vi "RS 485 IO.vi"(6 "Port":T1, 10 "Input in":T2={"Data"=[0, 0, 0, 0, 0, 0, 0, 0, 0, 0, 0, 0, 0, 0, 0, 0, 0, 0, 0, 0], "NumBytes"=0, "RS485_Cmd"=enum."Read", "Timeout (ms)"=0}) -> (3 "Input out":T3)   [LabVIEW 2015]
uses:
  RS485 In.ctl
  Serial Data In.ctl
  Port.ctl
  <vilib>/rvi/Emulation/niFpgaGetClockAttributes.vi
  <vilib>/rvi/Emulation/niFpgaSctlEmulationGetInTimedLoop.vi
  <vilib>/rvi/Emulation/niFpgaEmulationReportErrorSimple.vi
  <vilib>/rvi/eio/common/nirviEmuTemplateMethod_errors.vi
  <vilib>/rvi/Emulation/niFpgaCriticalErrorInLSC.vi
  <vilib>/eio/EIOMethodNode/EIOMethodNode.xnode
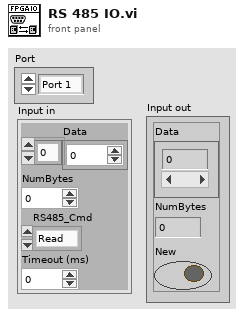
[diagram p1: front panel]
types:
  T1 = typedef "Port.ctl" = enum8{"Port 1", "Port 2", "Port 3", "Port 4", "None"}
  T2 = typedef "Serial Data In.ctl" = cluster{"Data":u8[], "NumBytes":i32, "RS485_Cmd":enum8{"Read", "Write", "Idle"}, "Timeout (ms)":i32}
  T3 = typedef "RS485 In.ctl" = cluster{"Data":u8[], "NumBytes":i32, "New":bool}
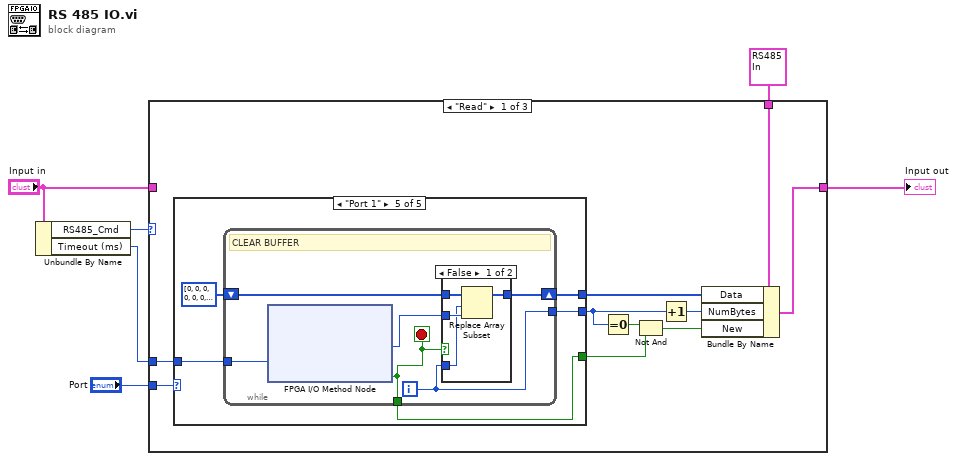
[diagram p0: block diagram]
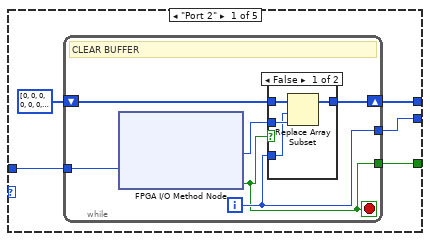
[diagram p2: hidden frame]
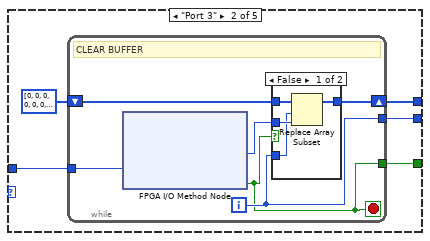
[diagram p4: hidden frame]
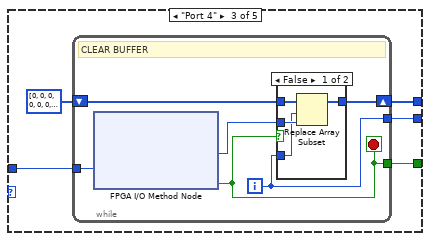
[diagram p6: hidden frame]
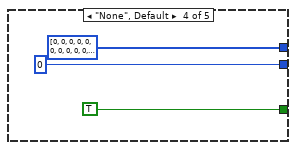
[diagram p8: hidden frame]
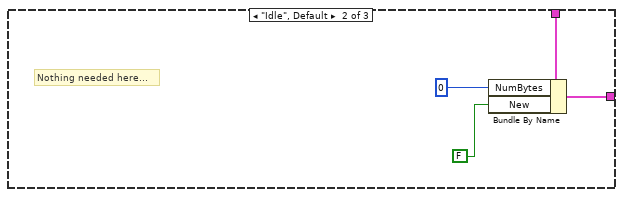
[diagram p10: hidden frame]
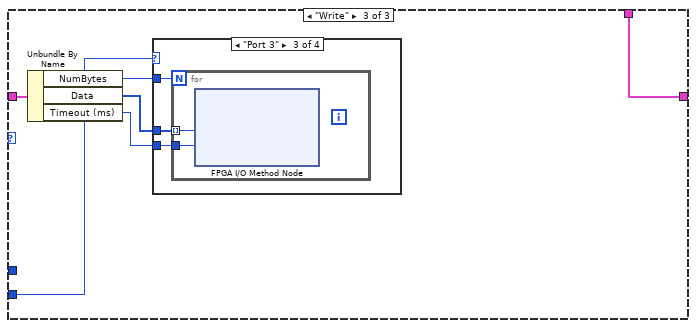
[diagram p11: hidden frame]
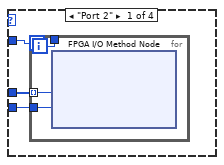
[diagram p12: hidden frame]
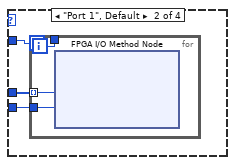
[diagram p13: hidden frame]
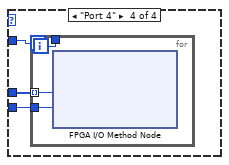
[diagram p14: hidden frame]
diagram:
  n1 = Unbundle By Name("Input in") -> ("RS485_Cmd"=w5:enum8{"Read", "Write", "Idle"}, "Timeout (ms)"=w6:i32)
  n2 = case shown="\"Read\"" w5 {
    tunnel: "Input in" -> [_ _ w93]
    tunnel: [w9 w84 w92] -> w2
    tunnel: w6 -> [w10 _ _]
    tunnel: "Port" -> [w7 _ w91]
    tunnel: T3 {"Data"=[0, 0, 0, 0, 0, 0, 0, 0, 0, 0, 0, 0, 0, 0, 0, 0, 0, 0, 0, 0, 0, 0, 0, 0, 0, 0, 0, 0, 0, 0, 0, 0, 0, 0, 0, 0, 0, 0, 0, 0, 0, 0, 0, 0, 0, 0, 0, 0, 0, 0, 0, 0, 0, 0, 0, 0, 0, 0, 0, 0, 0, 0, 0, 0, 0, 0, 0, 0, 0, 0, 0, 0, 0, 0, 0, 0, 0, 0, 0, 0, 0, 0, 0, 0, 0, 0, 0, 0, 0, 0, 0, 0, 0, 0, 0, 0, 0, 0, 0, 0, 0, 0, 0, 0, 0, 0, 0, 0, 0, 0, 0, 0, 0, 0, 0, 0, 0, 0, 0, 0, 0, 0, 0, 0, 0, 0, 0, 0, 0, 0, 0, 0, 0, 0, 0, 0, 0, 0, 0, 0, 0, 0, 0, 0, 0, 0, 0, 0, 0, 0, 0, 0, 0, 0, 0, 0, 0, 0, 0, 0, 0, 0, 0, 0, 0, 0, 0, 0, 0, 0, 0, 0, 0, 0, 0, 0, 0, 0, 0, 0, 0, 0, 0, 0, 0, 0, 0, 0, 0, 0, 0, 0, 0, 0, 0, 0, 0, 0, 0, 0], "NumBytes"=0, "New"=FALSE} ("Input out") -> [w8 w87 w92]
    frame "Read" {
      n3 = case shown="\"Port 1\"" w7 {
        tunnel: [w20 w36 w52 u8[] [0, 0, 0, 0, 0, 0, 0, 0, 0, 0, 0, 0, 0, 0, 0, 0, 0, 0, 0, 0, 0, 0, 0, 0, 0, 0, 0, 0, 0, 0, 0, 0, 0, 0, 0, 0, 0, 0, 0, 0, 0, 0, 0, 0, 0, 0, 0, 0, 0, 0, 0, 0, 0, 0, 0, 0, 0, 0, 0, 0, 0, 0, 0, 0, 0, 0, 0, 0, 0, 0, 0, 0, 0, 0, 0, 0, 0, 0, 0, 0, 0, 0, 0, 0, 0, 0, 0, 0, 0, 0, 0, 0, 0, 0, 0, 0, 0, 0, 0, 0, 0, 0, 0, 0, 0, 0, 0, 0, 0, 0, 0, 0, 0, 0, 0, 0, 0, 0, 0, 0, 0, 0, 0, 0, 0, 0, 0, 0, 0, 0, 0, 0, 0, 0, 0, 0, 0, 0, 0, 0, 0, 0, 0, 0, 0, 0, 0, 0, 0, 0, 0, 0, 0, 0, 0, 0, 0, 0, 0, 0, 0, 0, 0, 0, 0, 0, 0, 0, 0, 0, 0, 0, 0, 0, 0, 0, 0, 0, 0, 0, 0, 0, 0, 0, 0, 0, 0, 0, 0, 0, 0, 0, 0, 0, 0, 0, 0, 0, 0, 0] w71] -> w16
        tunnel: [w19 w35 w51 0 w70] -> w13
        tunnel: w10 -> [w18 w34 w50 _ w69]
        tunnel: [w17 w33 w49 TRUE ("Timed Out") w68] -> w12
        frame "Port 2" {
          n4 = while {
            shift-right: [w26] -> w20
            shift-left: u8[] [0, 0, 0, 0, 0, 0, 0, 0, 0, 0, 0, 0, 0, 0, 0, 0, 0, 0, 0, 0, 0, 0, 0, 0, 0, 0, 0, 0, 0, 0, 0, 0, 0, 0, 0, 0, 0, 0, 0, 0, 0, 0, 0, 0, 0, 0, 0, 0, 0, 0, 0, 0, 0, 0, 0, 0, 0, 0, 0, 0, 0, 0, 0, 0, 0, 0, 0, 0, 0, 0, 0, 0, 0, 0, 0, 0, 0, 0, 0, 0, 0, 0, 0, 0, 0, 0, 0, 0, 0, 0, 0, 0, 0, 0, 0, 0, 0, 0, 0, 0, 0, 0, 0, 0, 0, 0, 0, 0, 0, 0, 0, 0, 0, 0, 0, 0, 0, 0, 0, 0, 0, 0, 0, 0, 0, 0, 0, 0, 0, 0, 0, 0, 0, 0, 0, 0, 0, 0, 0, 0, 0, 0, 0, 0, 0, 0, 0, 0, 0, 0, 0, 0, 0, 0, 0, 0, 0, 0, 0, 0, 0, 0, 0, 0, 0, 0, 0, 0, 0, 0, 0, 0, 0, 0, 0, 0, 0, 0, 0, 0, 0, 0, 0, 0, 0, 0, 0, 0, 0, 0, 0, 0, 0, 0, 0, 0, 0, 0, 0, 0] -> [w27]
            tunnel: [w25] -> w19
            tunnel: w18 -> [w23]
            tunnel: [w22] -> w17
            i -> [w25]
            stop <- w22 stop-if-true
            # "CLEAR BUFFER"
            n5 = xnode "FPGA I/O Method Node"("Timeout (ms)"=w23) -> ("Data"=w24:u8, "Timed Out"=w22:bool)  [unwired: 1 in, 1 out]
            n6 = case shown="False" w22 {
              tunnel: w27 -> [w31 w32]
              tunnel: [w28 w32] -> w26
              tunnel: w24 -> [w30 _]
              tunnel: w25 -> [w29 _]
              frame False {
                n7 = Replace Array Subset(array=w31, new element=w30, index=w29) -> (w28:u8[])
              }
              frame True {
              }
            }
          }
        }
        frame "Port 3" {
          n8 = while {
            shift-right: [w42] -> w36
            shift-left: u8[] [0, 0, 0, 0, 0, 0, 0, 0, 0, 0, 0, 0, 0, 0, 0, 0, 0, 0, 0, 0, 0, 0, 0, 0, 0, 0, 0, 0, 0, 0, 0, 0, 0, 0, 0, 0, 0, 0, 0, 0, 0, 0, 0, 0, 0, 0, 0, 0, 0, 0, 0, 0, 0, 0, 0, 0, 0, 0, 0, 0, 0, 0, 0, 0, 0, 0, 0, 0, 0, 0, 0, 0, 0, 0, 0, 0, 0, 0, 0, 0, 0, 0, 0, 0, 0, 0, 0, 0, 0, 0, 0, 0, 0, 0, 0, 0, 0, 0, 0, 0, 0, 0, 0, 0, 0, 0, 0, 0, 0, 0, 0, 0, 0, 0, 0, 0, 0, 0, 0, 0, 0, 0, 0, 0, 0, 0, 0, 0, 0, 0, 0, 0, 0, 0, 0, 0, 0, 0, 0, 0, 0, 0, 0, 0, 0, 0, 0, 0, 0, 0, 0, 0, 0, 0, 0, 0, 0, 0, 0, 0, 0, 0, 0, 0, 0, 0, 0, 0, 0, 0, 0, 0, 0, 0, 0, 0, 0, 0, 0, 0, 0, 0, 0, 0, 0, 0, 0, 0, 0, 0, 0, 0, 0, 0, 0, 0, 0, 0, 0, 0] -> [w43]
            tunnel: [w41] -> w35
            tunnel: w34 -> [w39]
            tunnel: [w38] -> w33
            i -> [w41]
            stop <- w38 stop-if-true
            # "CLEAR BUFFER"
            n9 = xnode "FPGA I/O Method Node"("Timeout (ms)"=w39) -> ("Data"=w40:u8, "Timed Out"=w38:bool)  [unwired: 1 in, 1 out]
            n10 = case shown="False" w38 {
              tunnel: w43 -> [w47 w48]
              tunnel: [w44 w48] -> w42
              tunnel: w40 -> [w46 _]
              tunnel: w41 -> [w45 _]
              frame False {
                n11 = Replace Array Subset(array=w47, new element=w46, index=w45) -> (w44:u8[])
              }
              frame True {
              }
            }
          }
        }
        frame "Port 4" {
          n12 = while {
            shift-right: [w58] -> w52
            shift-left: u8[] [0, 0, 0, 0, 0, 0, 0, 0, 0, 0, 0, 0, 0, 0, 0, 0, 0, 0, 0, 0, 0, 0, 0, 0, 0, 0, 0, 0, 0, 0, 0, 0, 0, 0, 0, 0, 0, 0, 0, 0, 0, 0, 0, 0, 0, 0, 0, 0, 0, 0, 0, 0, 0, 0, 0, 0, 0, 0, 0, 0, 0, 0, 0, 0, 0, 0, 0, 0, 0, 0, 0, 0, 0, 0, 0, 0, 0, 0, 0, 0, 0, 0, 0, 0, 0, 0, 0, 0, 0, 0, 0, 0, 0, 0, 0, 0, 0, 0, 0, 0, 0, 0, 0, 0, 0, 0, 0, 0, 0, 0, 0, 0, 0, 0, 0, 0, 0, 0, 0, 0, 0, 0, 0, 0, 0, 0, 0, 0, 0, 0, 0, 0, 0, 0, 0, 0, 0, 0, 0, 0, 0, 0, 0, 0, 0, 0, 0, 0, 0, 0, 0, 0, 0, 0, 0, 0, 0, 0, 0, 0, 0, 0, 0, 0, 0, 0, 0, 0, 0, 0, 0, 0, 0, 0, 0, 0, 0, 0, 0, 0, 0, 0, 0, 0, 0, 0, 0, 0, 0, 0, 0, 0, 0, 0, 0, 0, 0, 0, 0, 0] -> [w59]
            tunnel: [w57] -> w51
            tunnel: w50 -> [w55]
            tunnel: [w54] -> w49
            i -> [w57]
            stop <- w54 stop-if-true
            # "CLEAR BUFFER"
            n13 = xnode "FPGA I/O Method Node"("Timeout (ms)"=w55) -> ("Data"=w56:u8, "Timed Out"=w54:bool)  [unwired: 1 in, 1 out]
            n14 = case shown="False" w54 {
              tunnel: w59 -> [w63 w64]
              tunnel: [w60 w64] -> w58
              tunnel: w56 -> [w62 _]
              tunnel: w57 -> [w61 _]
              frame False {
                n15 = Replace Array Subset(array=w63, new element=w62, index=w61) -> (w60:u8[])
              }
              frame True {
              }
            }
          }
        }
        frame "None", Default {
        }
        frame "Port 1" {
          n16 = while {
            shift-right: [w77] -> w71
            shift-left: u8[] [0, 0, 0, 0, 0, 0, 0, 0, 0, 0, 0, 0, 0, 0, 0, 0, 0, 0, 0, 0, 0, 0, 0, 0, 0, 0, 0, 0, 0, 0, 0, 0, 0, 0, 0, 0, 0, 0, 0, 0, 0, 0, 0, 0, 0, 0, 0, 0, 0, 0, 0, 0, 0, 0, 0, 0, 0, 0, 0, 0, 0, 0, 0, 0, 0, 0, 0, 0, 0, 0, 0, 0, 0, 0, 0, 0, 0, 0, 0, 0, 0, 0, 0, 0, 0, 0, 0, 0, 0, 0, 0, 0, 0, 0, 0, 0, 0, 0, 0, 0, 0, 0, 0, 0, 0, 0, 0, 0, 0, 0, 0, 0, 0, 0, 0, 0, 0, 0, 0, 0, 0, 0, 0, 0, 0, 0, 0, 0, 0, 0, 0, 0, 0, 0, 0, 0, 0, 0, 0, 0, 0, 0, 0, 0, 0, 0, 0, 0, 0, 0, 0, 0, 0, 0, 0, 0, 0, 0, 0, 0, 0, 0, 0, 0, 0, 0, 0, 0, 0, 0, 0, 0, 0, 0, 0, 0, 0, 0, 0, 0, 0, 0, 0, 0, 0, 0, 0, 0, 0, 0, 0, 0, 0, 0, 0, 0, 0, 0, 0, 0] -> [w78]
            tunnel: [w76] -> w70
            tunnel: w69 -> [w74]
            tunnel: [w73] -> w68
            i -> [w76]
            stop <- w73 stop-if-true
            # "CLEAR BUFFER"
            n17 = xnode "FPGA I/O Method Node"("Timeout (ms)"=w74) -> ("Data"=w75:u8, "Timed Out"=w73:bool)  [unwired: 1 in, 1 out]
            n18 = case shown="False" w73 {
              tunnel: w78 -> [w82 w83]
              tunnel: [w79 w83] -> w77
              tunnel: w75 -> [w81 _]
              tunnel: w76 -> [w80 _]
              frame False {
                n19 = Replace Array Subset(array=w82, new element=w81, index=w80) -> (w79:u8[])
              }
              frame True {
              }
            }
          }
        }
      }
      n20 = Equal To 0?(x=w13) -> (x = 0?=w14:bool)
      n21 = Not And(1:w12, 2:w14) -> (0:w11:bool)
      n22 = Increment(x=w13) -> (x+1=w15:i32)
      n23 = Bundle By Name(cluster=w8, "Data"=w16, "NumBytes"=w15, "New"=w11) -> (w9:T3)
    }
    frame "Idle", Default {
      # "Nothing needed here..."
      n24 = Bundle By Name(cluster=w87, "NumBytes"=0, "New"=FALSE) -> (w84:T3)
    }
    frame "Write" {
      n25 = Unbundle By Name(w93) -> ("NumBytes"=w90:i32, "Data"=w88:u8[], "Timeout (ms)"=w89:i32)
      n26 = case shown="\"Port 3\"" w91 {
        tunnel: w90 -> [w96 w102 w108 w113]
        tunnel: w88 -> [w95 w101 w107 w112]
        tunnel: w89 -> [w94 w100 w106 w111]
        frame "Port 2" {
          n27 = for {
            N: w96 -> [_]
            tunnel: w95 -> [w98] mode=indexing
            tunnel: w94 -> [w99]
            tunnel: [w97] -> _
            i -> [w97]
            n28 = xnode "FPGA I/O Method Node"("Data"=w98, "Timeout (ms)"=w99) -> ()  [unwired: 2 in, 3 out]
          }
        }
        frame "Port 1", Default {
          n29 = for {
            N: w102 -> [_]
            tunnel: w101 -> [w105] mode=indexing
            tunnel: w100 -> [w104]
            tunnel: [w103] -> _
            i -> [w103]
            n30 = xnode "FPGA I/O Method Node"("Data"=w105, "Timeout (ms)"=w104) -> ()  [unwired: 2 in, 3 out]
          }
        }
        frame "Port 3" {
          n31 = for {
            N: w108 -> [_]
            tunnel: w107 -> [w110] mode=indexing
            tunnel: w106 -> [w109]
            n32 = xnode "FPGA I/O Method Node"("Data"=w110, "Timeout (ms)"=w109) -> ()  [unwired: 2 in, 3 out]
          }
        }
        frame "Port 4" {
          n33 = for {
            N: w113 -> [_]
            tunnel: w112 -> [w116] mode=indexing
            tunnel: w111 -> [w115]
            tunnel: [w114] -> _
            i -> [w114]
            n34 = xnode "FPGA I/O Method Node"("Data"=w116, "Timeout (ms)"=w115) -> ()  [unwired: 2 in, 3 out]
          }
        }
      }
    }
  }
  "Input out" <- w2
